vi "OpenCamera.vi"(8 "error in (no error)":errorcluster, 11 "HamaCam in":refnum<class "HamaCam.lvclass">) -> (0 "error out":errorcluster, 3 "HamaCam out":refnum<class "HamaCam.lvclass">)   [LabVIEW 2023, in "HamaCam.lvlib" / "HamaCam.lvclass"]
uses:
  HamaCam.lvclass
  HamaCam.lvclass/HamaCam.ctl
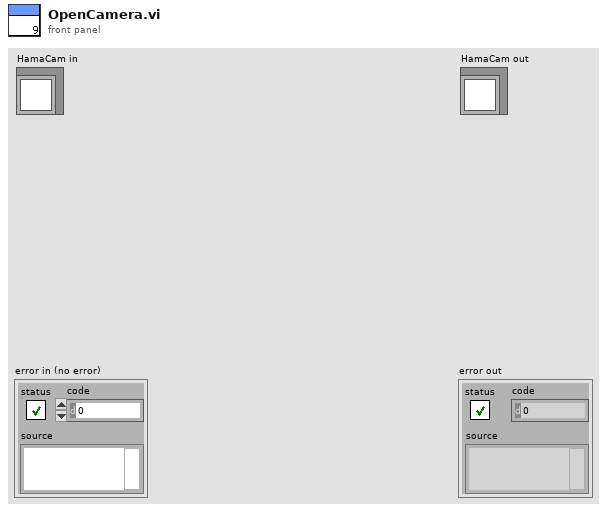
[diagram p1: front panel]
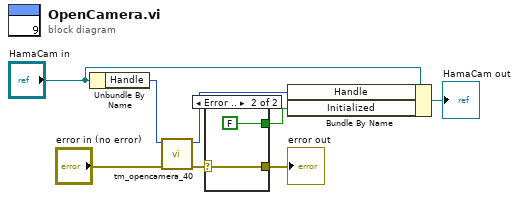
[diagram p0: block diagram]
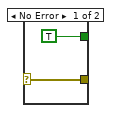
[diagram p2: hidden frame]
diagram:
  n1 = Unbundle By Name("HamaCam in") -> ("Handle"=w8:u32)
  n2 = call "tm_opencamera_40.vi"("error in (no error)"="error in (no error)", "Camera Index"=w8) -> ("error out"=w3:errorcluster, "Handle out"=w4:u32)  [unwired: 7 in, 1 out]
  n3 = case shown="Error .." w3 {
    selector: w3 -> [w10 w11]
    tunnel: [w10 w11] -> w2
    tunnel: [TRUE ("CurrentState.Initialized") FALSE ("CurrentState.Initialized")] -> w1
    frame No Error {
    }
    frame Error {
    }
  }
  "error out" <- w2
  n4 = Bundle By Name(cluster="HamaCam in", "Handle"=w4, "Initialized"=w1) -> (→"HamaCam out":refnum<class "HamaCam.lvclass">)
